vi "EminemDashRead.vi"(8 "error in (no error)":errorcluster) -> (0 "error out":errorcluster)   [LabVIEW 2023]
uses:
  EminemGlobals.vi
  <vilib>/Rock Robotics/Network Tables/NT Read Number.vi
  <vilib>/Rock Robotics/Network Tables/NT Write Number.vi
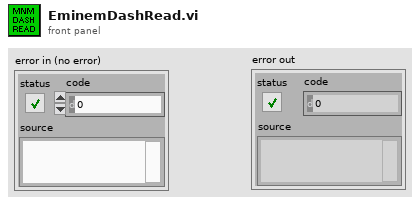
[diagram p1: front panel]
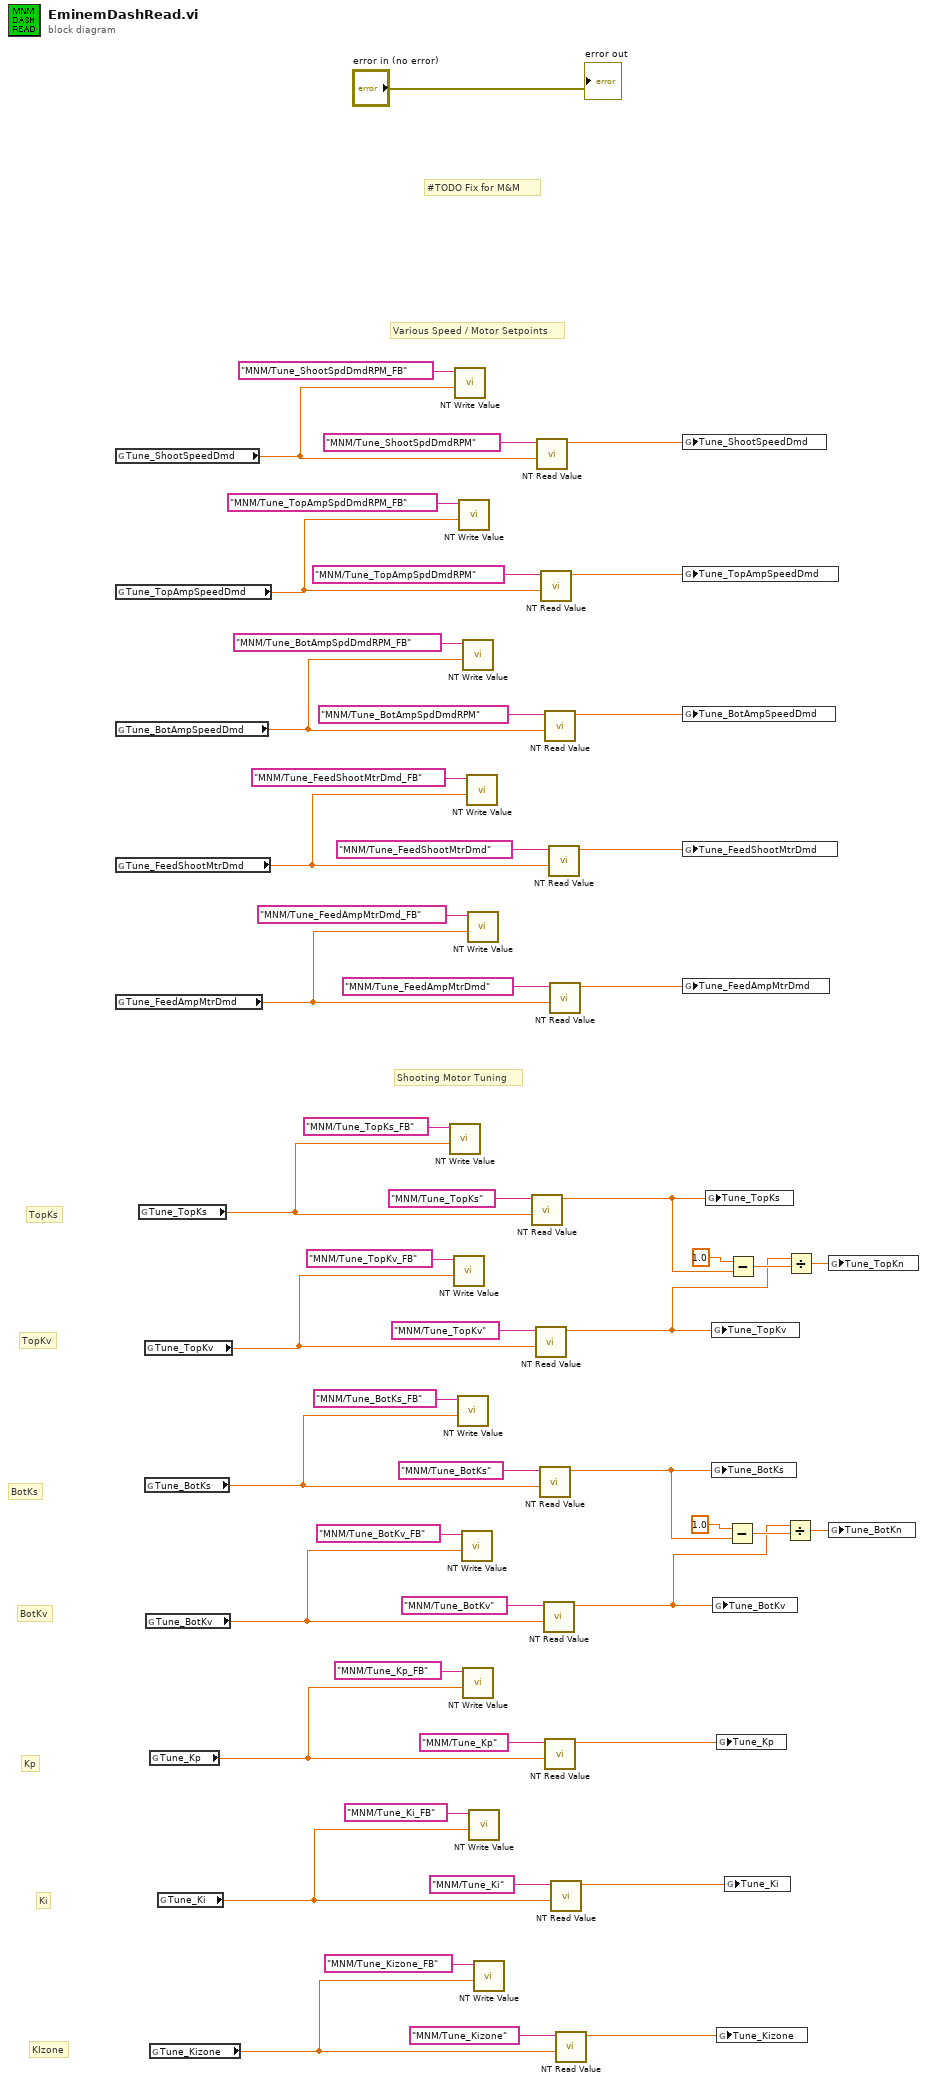
[diagram p0: block diagram]
diagram:
  # "KIzone"
  # "Ki"
  # "Kp"
  # "BotKv"
  # "BotKs"
  # "TopKv"
  # "TopKs"
  # "Shooting Motor Tuning"
  # "Various Speed / Motor Setpoints"
  # "#TODO Fix for M&M"
  n1 = global read "EminemGlobals.vi" "Tune_ShootSpeedDmd"() -> (w52:dbl)
  n2 = global read "EminemGlobals.vi" "Tune_TopAmpSpeedDmd"() -> (w37:dbl)
  n3 = global read "EminemGlobals.vi" "Tune_BotAmpSpeedDmd"() -> (w36:dbl)
  n4 = global read "EminemGlobals.vi" "Tune_FeedShootMtrDmd"() -> (w35:dbl)
  n5 = global read "EminemGlobals.vi" "Tune_FeedAmpMtrDmd"() -> (w38:dbl)
  n6 = global read "EminemGlobals.vi" "Tune_TopKs"() -> (w32:dbl)
  n7 = global read "EminemGlobals.vi" "Tune_TopKv"() -> (w21:dbl)
  n8 = global read "EminemGlobals.vi" "Tune_BotKs"() -> (w20:dbl)
  n9 = global read "EminemGlobals.vi" "Tune_BotKv"() -> (w19:dbl)
  n10 = global read "EminemGlobals.vi" "Tune_Kp"() -> (w22:dbl)
  n11 = global read "EminemGlobals.vi" "Tune_Kizone"() -> (w11:dbl)
  n12 = global read "EminemGlobals.vi" "Tune_Ki"() -> (w15:dbl)
  n13 = call-poly <vilib>:"NT Write Value.vi"("value"=w32, "name"="MNM/Tune_TopKs_FB") -> ()  [unwired: 9 in, 1 out]
  n14 = call-poly <vilib>:"NT Write Value.vi"("value"=w21, "name"="MNM/Tune_TopKv_FB") -> ()  [unwired: 9 in, 1 out]
  n15 = call-poly <vilib>:"NT Write Value.vi"("value"=w52, "name"="MNM/Tune_ShootSpdDmdRPM_FB") -> ()  [unwired: 9 in, 1 out]
  n16 = call-poly <vilib>:"NT Write Value.vi"("value"=w20, "name"="MNM/Tune_BotKs_FB") -> ()  [unwired: 9 in, 1 out]
  n17 = call-poly <vilib>:"NT Write Value.vi"("value"=w37, "name"="MNM/Tune_TopAmpSpdDmdRPM_FB") -> ()  [unwired: 9 in, 1 out]
  n18 = call-poly <vilib>:"NT Write Value.vi"("value"=w19, "name"="MNM/Tune_BotKv_FB") -> ()  [unwired: 9 in, 1 out]
  n19 = call-poly <vilib>:"NT Write Value.vi"("value"=w36, "name"="MNM/Tune_BotAmpSpdDmdRPM_FB") -> ()  [unwired: 9 in, 1 out]
  n20 = call-poly <vilib>:"NT Write Value.vi"("value"=w22, "name"="MNM/Tune_Kp_FB") -> ()  [unwired: 9 in, 1 out]
  n21 = call-poly <vilib>:"NT Write Value.vi"("value"=w35, "name"="MNM/Tune_FeedShootMtrDmd_FB") -> ()  [unwired: 9 in, 1 out]
  n22 = call-poly <vilib>:"NT Write Value.vi"("value"=w38, "name"="MNM/Tune_FeedAmpMtrDmd_FB") -> ()  [unwired: 9 in, 1 out]
  n23 = call-poly <vilib>:"NT Write Value.vi"("value"=w15, "name"="MNM/Tune_Ki_FB") -> ()  [unwired: 9 in, 1 out]
  n24 = call-poly <vilib>:"NT Write Value.vi"("value"=w11, "name"="MNM/Tune_Kizone_FB") -> ()  [unwired: 9 in, 1 out]
  n25 = call-poly <vilib>:"NT Read Value.vi"("default value"=w32, "name"="MNM/Tune_TopKs") -> ("value"=w9:dbl)  [unwired: 7 in, 2 out]
  n26 = call-poly <vilib>:"NT Read Value.vi"("default value"=w21, "name"="MNM/Tune_TopKv") -> ("value"=w7:dbl)  [unwired: 7 in, 2 out]
  n27 = call-poly <vilib>:"NT Read Value.vi"("default value"=w52, "name"="MNM/Tune_ShootSpdDmdRPM") -> ("value"=w51:dbl)  [unwired: 7 in, 2 out]
  n28 = call-poly <vilib>:"NT Read Value.vi"("default value"=w20, "name"="MNM/Tune_BotKs") -> ("value"=w1:dbl)  [unwired: 7 in, 2 out]
  n29 = call-poly <vilib>:"NT Read Value.vi"("default value"=w37, "name"="MNM/Tune_TopAmpSpdDmdRPM") -> ("value"=w42:dbl)  [unwired: 7 in, 2 out]
  n30 = call-poly <vilib>:"NT Read Value.vi"("default value"=w19, "name"="MNM/Tune_BotKv") -> ("value"=w2:dbl)  [unwired: 7 in, 2 out]
  n31 = call-poly <vilib>:"NT Read Value.vi"("default value"=w36, "name"="MNM/Tune_BotAmpSpdDmdRPM") -> ("value"=w41:dbl)  [unwired: 7 in, 2 out]
  n32 = call-poly <vilib>:"NT Read Value.vi"("default value"=w22, "name"="MNM/Tune_Kp") -> ("value"=w23:dbl)  [unwired: 7 in, 2 out]
  n33 = call-poly <vilib>:"NT Read Value.vi"("default value"=w35, "name"="MNM/Tune_FeedShootMtrDmd") -> ("value"=w40:dbl)  [unwired: 7 in, 2 out]
  n34 = call-poly <vilib>:"NT Read Value.vi"("default value"=w38, "name"="MNM/Tune_FeedAmpMtrDmd") -> ("value"=w39:dbl)  [unwired: 7 in, 2 out]
  n35 = call-poly <vilib>:"NT Read Value.vi"("default value"=w15, "name"="MNM/Tune_Ki") -> ("value"=w16:dbl)  [unwired: 7 in, 2 out]
  n36 = call-poly <vilib>:"NT Read Value.vi"("default value"=w11, "name"="MNM/Tune_Kizone") -> ("value"=w12:dbl)  [unwired: 7 in, 2 out]
  n37 = global write "EminemGlobals.vi" "Tune_ShootSpeedDmd"(w51) -> ()
  n38 = global write "EminemGlobals.vi" "Tune_TopAmpSpeedDmd"(w42) -> ()
  n39 = global write "EminemGlobals.vi" "Tune_BotAmpSpeedDmd"(w41) -> ()
  n40 = global write "EminemGlobals.vi" "Tune_FeedShootMtrDmd"(w40) -> ()
  n41 = global write "EminemGlobals.vi" "Tune_FeedAmpMtrDmd"(w39) -> ()
  n42 = global write "EminemGlobals.vi" "Tune_TopKs"(w9) -> ()
  n43 = global write "EminemGlobals.vi" "Tune_TopKv"(w7) -> ()
  n44 = global write "EminemGlobals.vi" "Tune_BotKs"(w1) -> ()
  n45 = global write "EminemGlobals.vi" "Tune_BotKv"(w2) -> ()
  n46 = global write "EminemGlobals.vi" "Tune_Kp"(w23) -> ()
  n47 = global write "EminemGlobals.vi" "Tune_Kizone"(w12) -> ()
  n48 = global write "EminemGlobals.vi" "Tune_Ki"(w16) -> ()
  n49 = Subtract(x=1.0, y=w1) -> (x-y=w4:dbl)
  n50 = Subtract(x=1.0, y=w9) -> (x-y=w8:dbl)
  n51 = Divide(x=w2, y=w4) -> (x/y=w3:dbl)
  n52 = Divide(x=w7, y=w8) -> (x/y=w6:dbl)
  n53 = global write "EminemGlobals.vi" "Tune_TopKn"(w6) -> ()
  n54 = global write "EminemGlobals.vi" "Tune_BotKn"(w3) -> ()
  "error out" <- "error in (no error)"
